vi "sensor config set label v2.vi"(7 "str_length":i32, 9 "label_str":string, 10 "label_string":u32(ring) items=["CONFIG_V2_STRING_LABEL_0", "CONFIG_V2_STRING_LABEL_1", "CONFIG_V2_STRING_LABEL_2", "CONFIG_V2_STRING_LOCATION", "CONFIG_V2_STRING_TIMEZONE", "CONFIG_V2_STRING_BUTTON_EVENT_0", "CONFIG_V2_STRING_BUTTON_EVENT_1", "CONFIG_V2_STRING_BUTTON_EVENT_2", "CONFIG_V2_STRING_BUTTON_EVENT_3", "CONFIG_V2_STRING_TIMEZONE_OFFSET", "CONFIG_V2_STRING_LAST_VALUE"], 11 "h":u32) -> (2 "function return":i32, 3 "h out":u32)   [LabVIEW 2019, in "apdm.lvlib"]
doc: "APDM_EXPORT int apdm_sensor_config_set_label_v2(apdm_device_handle_t h, const config_v2_string_t label_string, const char label_str[24], const int str_length);"
uses:
  apdm.lvlib
  Lee Lab/CP FES Walking 2018/Code/Working/LabVIEW/apdm.dll
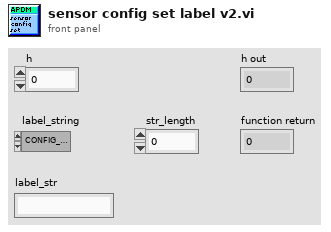
[diagram p1: front panel]
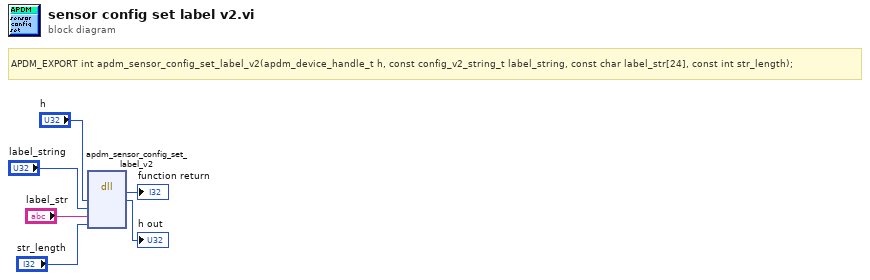
[diagram p0: block diagram]
diagram:
  # "APDM_EXPORT int apdm_sensor_config_set_label_v2(apdm_device_handle_t h, const config_v2_string_t label_string, const char label_str[24], const int str_length);"
  n1 = dll-call lib="C:/Users/jfalesi/Dropbox/Lee Lab/CP FES Walking 2018/Code/Working/LabVIEW/apdm.*" fn="apdm_sensor_config_set_label_v2"("h"="h", "label_string"="label_string", "label_str"="label_str", "str_length"="str_length") -> (→"function return":i32, "h"=→"h out":u32)  [unwired: 6 in, 2 out]
